vi "Untitled 2.vi"(0 "Offset":dbl, 2 "Reset Signal":bool, 5 "Frequency":dbl=10.1, 7 "Amplitude":dbl=1.0, 9 "Phase":dbl, 11 "error in (no error)":errorcluster) -> (4 "Sine":dynamicdata(graph), 15 "error out":errorcluster)   [LabVIEW 2021]
doc: "Simulates a sine wave, square wave, triangle wave, sawtooth wave, or noise signal.\n--------------------\n\nThis Express VI is configured as follows:\n\nSignal Type: Sine\nFrequency: 10.1 Hz\nAmplitude: 1\nPhase: 0\nOffset: 0\nSampling Rate: 1000 Hz\nNumber of Samples: 100 (Automatic)\nTiming: Run as fast as possible\nTimestamps: Relative"
panel:
  in  "Trials":i32=1
  in  "Seed Number":dbl=-1.0
  in  "Noise amplitude":dbl=0.6
  in  "Duty Cycle (%)":dbl=50.0
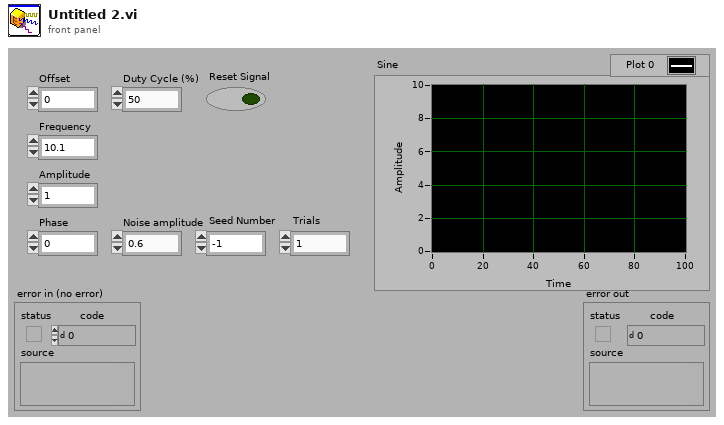
[diagram p1: front panel]
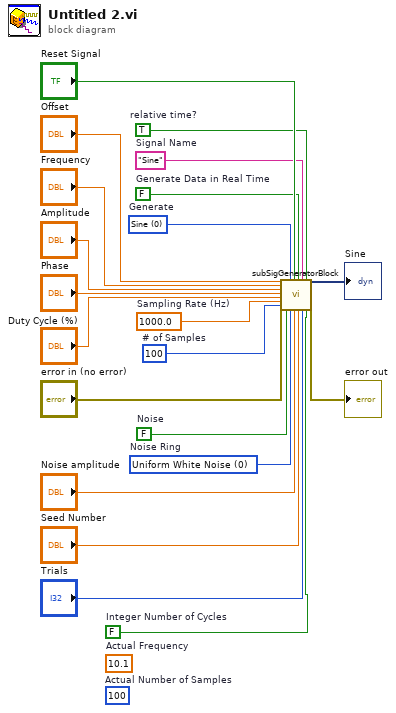
[diagram p0: block diagram]
diagram:
  (unwired) 10.1  # Actual Frequency
  (unwired) 100  # Actual Number of Samples
  w1 = FALSE  # Integer Number of Cycles
  w5 = u16 0 items=["Uniform White Noise", "Gaussian White Noise", "Periodic Random Noise", "Gamma Noise", "Poisson Noise", "Binomial Noise", "Bernoulli Noise", "MLS Sequence "]  # Noise Ring
  w6 = FALSE  # Noise
  w9 = TRUE  # relative time?
  w10 = "Sine"  # Signal Name
  w11 = FALSE  # Generate Data in Real Time
  w13 = u16 0 items=["Sine", "Square", "Triangle", "Sawtooth", "DC"]  # Generate
  w15 = 100  # # of Samples
  w17 = 1000.0  # Sampling Rate (Hz)
  n1 = call <vilib>:"subSigGeneratorBlock.vi"("Offset"="Offset", "Frequency"="Frequency", "Amplitude"="Amplitude", "Phase"="Phase", "Duty Cycle (%)"="Duty Cycle (%)", "Sampling Rate (Hz)"=w17, "# of Samples"=w15, "error in (no error)"="error in (no error)", "Noise"=w6, "Generate"=w13, "Noise Ring"=w5, "Reset Signal"="Reset Signal", "Noise Amplitude"="Noise amplitude", "Generate Data in Real Time"=w11, "Seed Number"="Seed Number", "Signal Name"=w10, "trials"="Trials", "relative time?"=w9, "Integer Number of Cycles"=w1) -> ("Signal"=→"Sine":dynamicdata, "error out"=→"error out":errorcluster)  [unwired: 7 in]
